vi "TCPIP_main_global.vi"() -> ()   [LabVIEW 2010]
panel:
  in  "Send":string
  out "END":bool
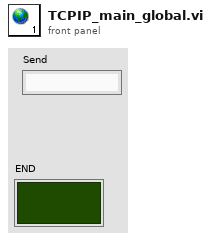
[diagram p1: front panel]
diagram:
